vi "Data Storage.vi"(9 "Time Out In ms":i32=-1, 10 "Data In":T1, 11 "1D U16 Group With ID DVR Queue in":refnum<class "2D U16 Group With ID DVR Queue.lvclass">) -> (1 "Time Out":bool, 3 "1D U16 Group With ID DVR Queue out":refnum<class "2D U16 Group With ID DVR Queue.lvclass">)   [LabVIEW 2019, in "2D U16 Group With ID DVR Queue.lvclass"]
uses:
  2D U16 Group With ID DVR Queue.lvclass
  Type Def/Data Type.ctl
  2D U16 Group With ID DVR Queue.lvclass/2D U16 Group With ID DVR Queue.ctl
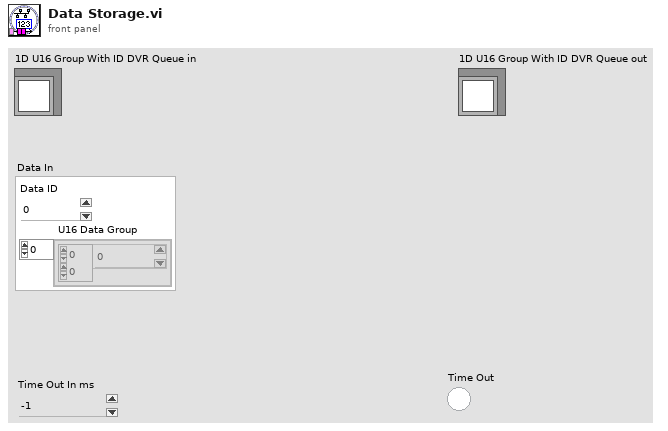
[diagram p1: front panel]
types:
  T1 = typedef "Data Type.ctl" = cluster{"Data ID":i64, "U16 Data Group":cluster{"Array":u16[][]}[]}
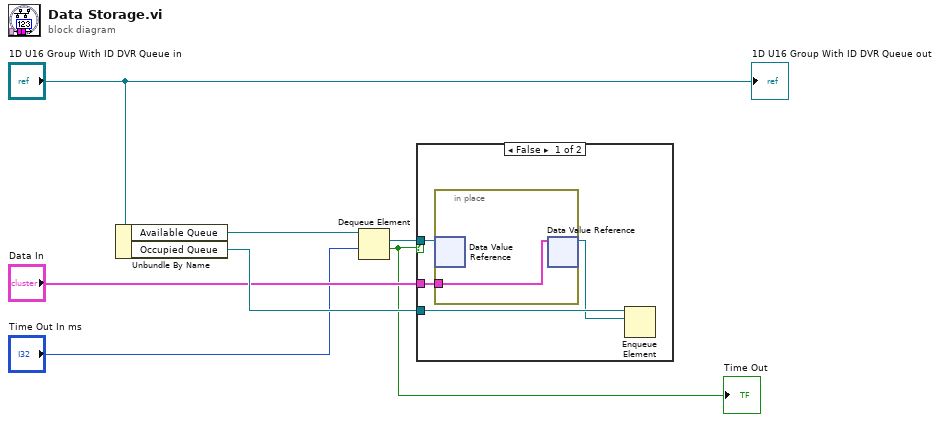
[diagram p0: block diagram]
diagram:
  n1 = Unbundle By Name("1D U16 Group With ID DVR Queue in") -> ("Available Queue"=w4:refnum<queue>, "Occupied Queue"=w7:refnum<queue>)
  n2 = Dequeue Element(queue=w4, timeout in ms (-1)="Time Out In ms") -> (element=w3:refnum<data-value>, timed out?=w2:bool)  [unwired: 1 in, 2 out]
  "Time Out" <- w2
  n3 = case shown="False" w2 {
    tunnel: w3 -> [w11 _]
    tunnel: w7 -> [w10 _]
    tunnel: "Data In" -> [w8 _]
    frame False {
      n4 = in-place {
        in-place-border: w8 -> [w12]
        n5 = in-place-dvr #1(w11) -> ()  [unwired: 2 out]
        n6 = in-place-dvr #1(w12) -> (w9:refnum<data-value>)  [unwired: 1 out]
      }
      n7 = Enqueue Element(queue=w10, element=w9) -> ()  [unwired: 2 in, 3 out]
    }
    frame True {
    }
  }
  "1D U16 Group With ID DVR Queue out" <- "1D U16 Group With ID DVR Queue in"
